vi "Get 1D I64.vi"(5 "format string (%_20f)":string="%_20f", 7 "key description":string, 8 "sections":string[](array[string]), 9 "numeric":i64[](array[numeric]), 11 "info data":string) -> (0 "sections out":string[](array[string]), 2 "value":i64[](array[numeric]), 3 "info data out":string)   [LabVIEW 2013, in "infolib.lvlib"]
doc: "Add a new numeric key to Info Data string. If section exists in Info Data string, inserts key into this section."
uses:
  infolib.lvlib
  Get 2D I64.vi
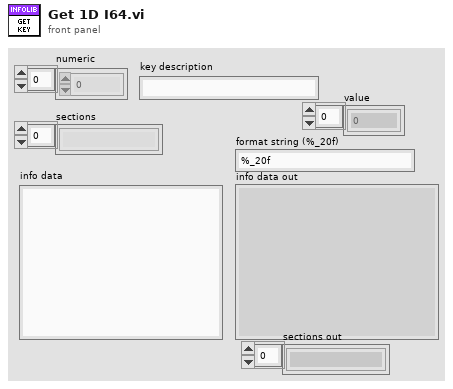
[diagram p1: front panel]
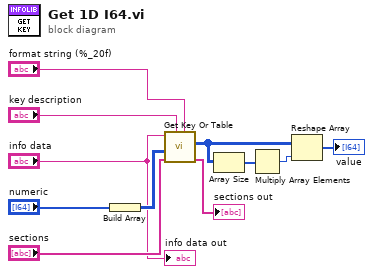
[diagram p0: block diagram]
diagram:
  n1 = Build Array("numeric") -> (w9:i64[][])
  n2 = call-poly "Get Key Or Table.vi"("format string (%_20f)"="format string (%_20f)", "key description"="key description", "sections"="sections", "numeric"=w9, "info data"="info data") -> ("sections out"=→"sections out":string[], "value"=w2:i64[][])  [unwired: 4 in, 1 out]
  n3 = Array Size(array=w2) -> (size(s)=w3:i32[])
  n4 = Multiply Array Elements(1:w3) -> (0:w4:i32)
  n5 = Reshape Array(w2, w4) -> (→"value":i64[])
  "info data out" <- "info data"
